vi "threshhold rowcol sums.vi"(8 "Row(T)/Col(F)":bool, 10 "Threshold":dbl=8.0 format="%#_13g", 11 "Pixels":u8[][](array[numeric])) -> (1 "last row/col":i32, 2 "middle row/col":i32, 3 "first row/col":i32)   [LabVIEW 2017]
doc: "Sums up the pixels values of each row or column. Then finds the first and last row/column that is above a threshold, as well as the middle row/column."
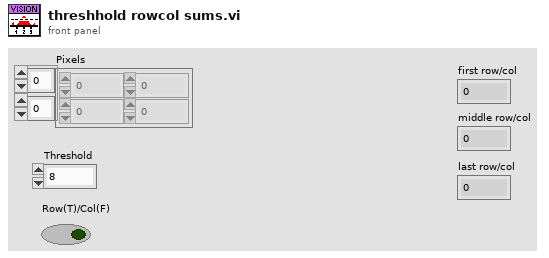
[diagram p1: front panel]
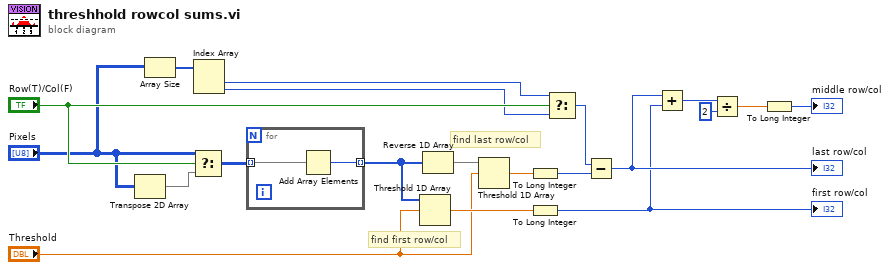
[diagram p0: block diagram]
diagram:
  # "find last row/col"
  # "find first row/col"
  n1 = Transpose 2D Array(2D array="Pixels") -> (transposed array=w9:u8[][])
  n2 = Array Size(array="Pixels") -> (size(s)=w4:i32[])
  n3 = Select(t="Pixels", s="Row(T)/Col(F)", f=w9) -> (s? t:f=w8:u8[][])
  n4 = Index Array(array=w4) -> (element #1=w2:i32, element #2=w1:i32)  [unwired: 2 in]
  n5 = for {
    tunnel: w8 -> [w22] mode=indexing
    tunnel: [w21] -> w16 mode=indexing
    n6 = Add Array Elements(numeric array=w22) -> (sum=w21:u8)
  }
  n7 = Threshold 1D Array(2:"Threshold", 3:w16) -> (0:w18:dbl)  [unwired: 1 in]
  n8 = Reverse 1D Array(array=w16) -> (reversed array=w19:u8[])
  n9 = Threshold 1D Array(2:"Threshold", 3:w19) -> (0:w17:dbl)  [unwired: 1 in]
  n10 = To Long Integer(number=w17) -> (32bit integer=w20:i32)
  n11 = To Long Integer(number=w18) -> (32bit integer=w14:i32)
  "first row/col" <- w14
  n12 = Select(t=w2, s="Row(T)/Col(F)", f=w1) -> (s? t:f=w6:i32)
  n13 = Subtract(x=w6, y=w20) -> (x-y=w15:i32)
  "last row/col" <- w15
  n14 = Add(x=w15, y=w14) -> (x+y=w13:i32)
  n15 = Divide(x=w13, y=2) -> (x/y=w11:dbl)
  n16 = To Long Integer(number=w11) -> (32bit integer=→"middle row/col":i32)
